vi "MTS_SetGraphScales.vi"(5 "Pixels":u16[](array[numeric]), 6 "Axis":enum32{"x-y", "x-z", "y-z"}(ring), 7 "Picture Size":dbl[](array[numeric]), 8 "error in (no error)":errorcluster, 10 "Upper Left":T1, 11 "Image":refnum<vi>) -> (0 "error out":errorcluster)   [LabVIEW 2010]
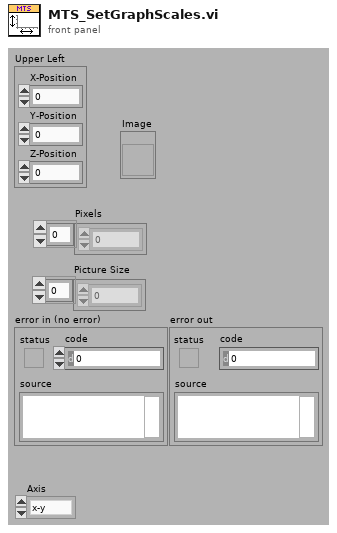
[diagram p1: front panel]
types:
  T1 = cluster{"X-Position":dbl, "Y-Position":dbl, "Z-Position":dbl}
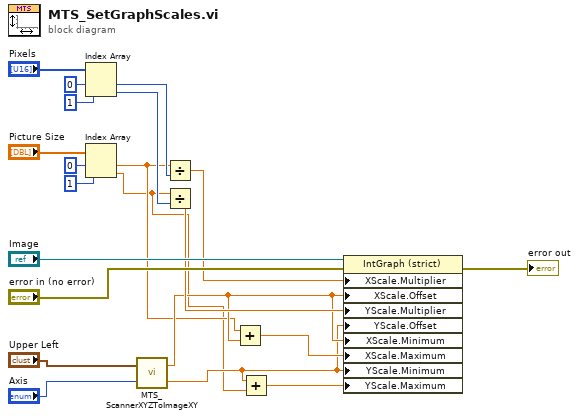
[diagram p0: block diagram]
diagram:
  n1 = Index Array(array="Pixels", index #1=0 ("index"), index #2=1 ("index")) -> (element #1=w12:u16, element #2=w10:u16)
  n2 = Index Array(array="Picture Size", index #1=0 ("index"), index #2=1 ("index")) -> (element #1=w5:dbl, element #2=w2:dbl)
  n3 = call "MTS_ScannerXYZToImageXY.vi"("Axis"="Axis", "Scanner XYZ"="Upper Left") -> ("Image Y"=w3:dbl, "Image X"=w6:dbl)
  n4 = Divide(x=w5, y=w12) -> (x/y=w11:dbl)
  n5 = Divide(x=w2, y=w10) -> (x/y=w9:dbl)
  n6 = Add(x=w5, y=w6) -> (x+y=w4:dbl)
  n7 = Add(x=w3, y=w2) -> (x+y=w1:dbl)
  n8 = property on="Property Node" class="IntGraph (strict)"(reference="Image", error in="error in (no error)", "XScale.Multiplier"=w11, "XScale.Offset"=w6, "YScale.Multiplier"=w9, "YScale.Offset"=w3, "XScale.Minimum"=w6, "XScale.Maximum"=w4, "YScale.Minimum"=w3, "YScale.Maximum"=w1) -> (error out=→"error out":errorcluster)  [unwired: 1 out]
